vi "Get Mode Code.vi"(8 "error in":errorcluster, 11 "message in":T1 format="%.0x") -> (0 "error out":errorcluster, 2 "mode code":u16, 3 "message out":T1 format="%.0x")   [LabVIEW 2020, in "Ballard MIL-STD-1553 Scripting.lvlib"]
uses:
  Ballard MIL-STD-1553 Scripting.lvlib
  Constants.vi
  <vilib>/NI VeriStand/Custom Device API/Custom Device API.lvlib
  <vilib>/NI VeriStand/Custom Device API/Get Item Property (U16).vi
  <vilib>/NI VeriStand/Custom Device API/Custom Device Item Ref.ctl
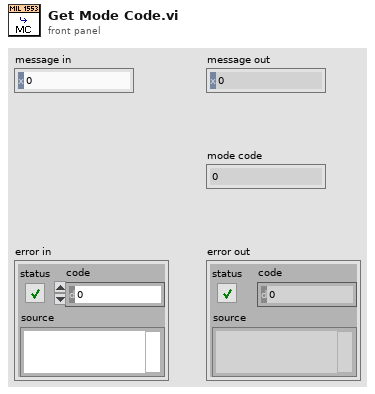
[diagram p1: front panel]
types:
  T1 = typedef "Custom Device API.lvlib/Custom Device Item Ref.ctl" = u64
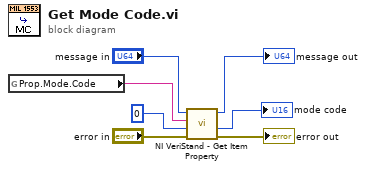
[diagram p0: block diagram]
diagram:
  n1 = global read "Constants.vi" "Prop.Mode.Code"() -> (w3:string)
  n2 = call-poly <vilib>:"NI VeriStand - Get Item Property.vi"("error in (no error)"="error in", "Default Value"=u16 0 ("number of words"), "Property Name"=w3, "Item Ref in"="message in") -> ("error out"=→"error out":errorcluster, "Value"=→"mode code":u16, "Item Ref out"=→"message out":T1)  [unwired: 4 in, 1 out]
